vi "Test 1 Get Next State from Node.vi"(8 "error in (no error)":errorcluster, 11 "Test Case In":refnum<class "Day 8 Test.lvclass">) -> (0 "error out":errorcluster, 3 "Test Case Out":refnum<class "Day 8 Test.lvclass">)   [LabVIEW 2020, in "Day 8 Test.lvclass"]
uses:
  Day 8 Test.lvclass
  C:/Program Files (x86)/National Instruments/LabVIEW 2020/vi.lib/Astemes/LUnit/Test Case.lvclass
  <vilib>/Astemes/LUnit/Test Case.lvclass/Test Case.ctl
  4993e8ee-a06a-463a-9684-69129f64d5ce.vi
  <vilib>/Astemes/LUnit/Append Pass Result.vi
  <vilib>/Astemes/LUnit/Append Fail Result.vi
  <vilib>/Astemes/LUnit/Describe Comparison.vi
  <vilib>/Astemes/LUnit/Compare Variants.vi
  <vilib>/Astemes/LUnit/Variant to string.vi
  <vilib>/Utility/Data Type/Get Type Information.vi
  <vilib>/Utility/LVClass/Get LV Class Name.vi
  Day 8 Test.lvclass/Day 8 Test.ctl
  Network/Network.lvclass
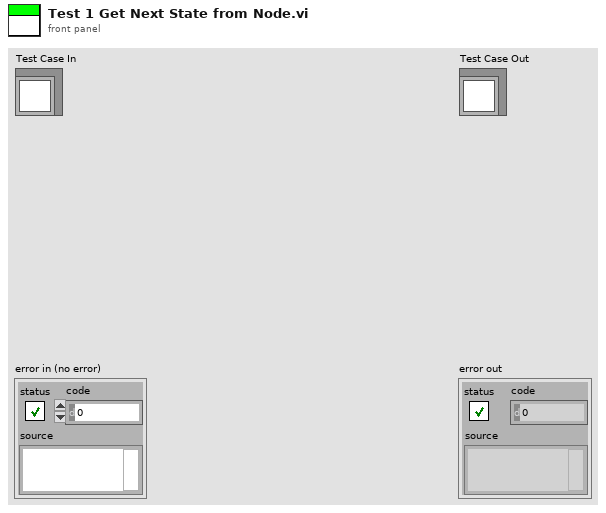
[diagram p1: front panel]
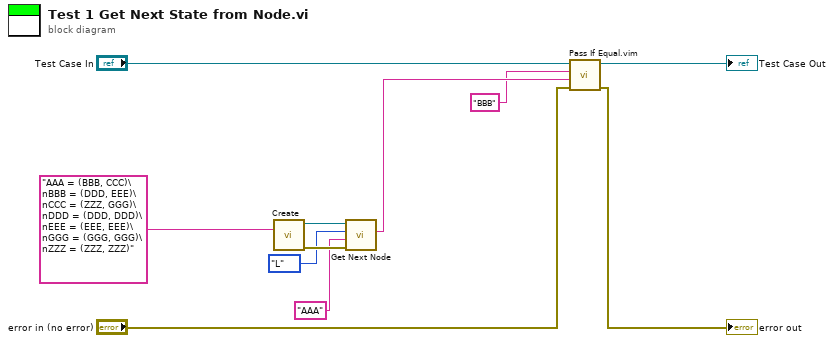
[diagram p0: block diagram]
diagram:
  n1 = call "Create.vi"("Input"="AAA = (BBB, CCC)\nBBB = (DDD, EEE)\nCCC = (ZZZ, GGG)\nDDD = (DDD, DDD)\nEEE = (EEE, EEE)\nGGG = (GGG, GGG)\nZZZ = (ZZZ, ZZZ)") -> ("error out"=w6:errorcluster, "Network"=w2:refnum<class "Network.lvclass">)  [unwired: 9 in]
  n2 = call "Get Next Node.vi"("error in (no error)"=w6, "State"="AAA", "Direction"=enum16{"L", "R"}."L", "Network in"=w2) -> ("Node"=w4:string)  [unwired: 5 in, 2 out]
  n3 = call "Pass If Equal.vim"("error in (no error)"="error in (no error)", "Actual"=w4, "Expected"="BBB" ("Node"), "LUnit Test Case In"="Test Case In") -> ("error out"=→"error out":errorcluster, "LUnit Test Case Out"=→"Test Case Out":refnum<class "Day 8 Test.lvclass">)  [unwired: 6 in]
